vi "Process_TCP_Host.vi"(0 "Q_TCP_Cmd_IN":refnum<queue>, 1 "Q_TCP_Cmd_Err_IN":errorcluster, 2 "Q_GetPacket_IN":refnum<queue>, 3 "Q_GetPacket_Err_IN":errorcluster, 4 "Notifier_IN":refnum<notifier>, 5 "Notifier_Err_IN":errorcluster, 8 "PortNumber":u16=25534, 10 "IP Addr":string) -> (14 "Q_TCP_Cmd_OUT":refnum<queue>, 15 "Q_TCP_Cmd_Err_OUT":errorcluster, 16 "Q_GetPacket_OUT":refnum<queue>, 17 "Q_GetPacket_Err_OUT":errorcluster)   [LabVIEW 2023]
uses:
  HOST_GLOBAL.vi
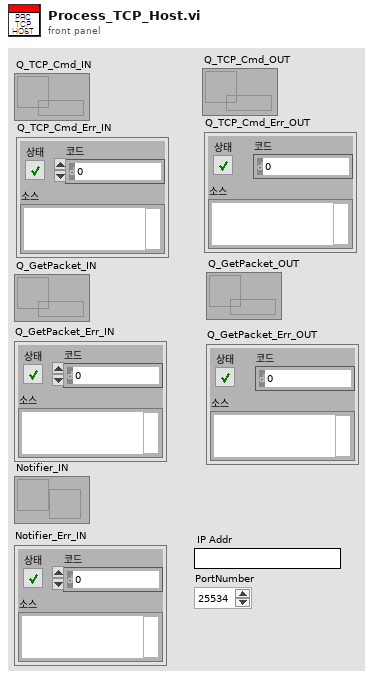
[diagram p1: front panel]
types:
  T1 = enum16{"Standard", "Buffered", "CRLF", "Immediate"}
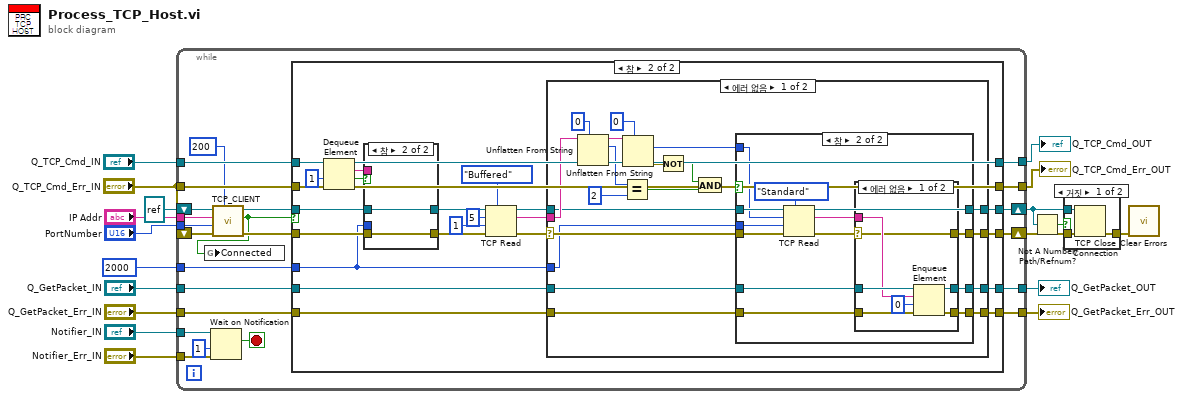
[diagram p0: block diagram]
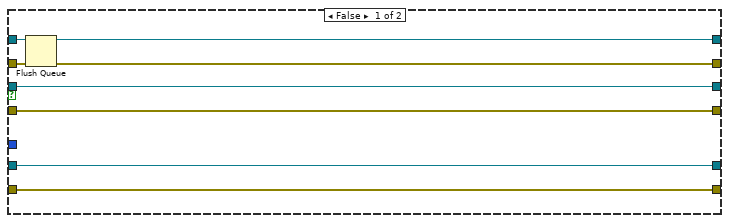
[diagram p3: hidden frame]
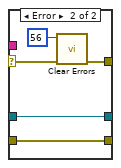
[diagram p5: hidden frame]
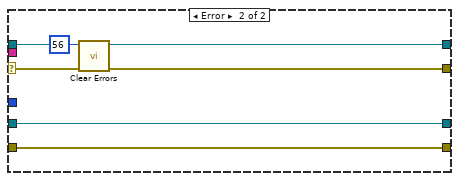
[diagram p6: hidden frame]
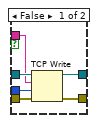
[diagram p7: hidden frame]
diagram:
  n1 = while {
    tunnel: "PortNumber" -> [w38]
    tunnel: "IP Addr" -> [w37]
    shift-right: [w23] -> w2
    shift-left: "Q_TCP_Cmd_Err_IN" -> [w41]
    shift-right: [w24] -> w1
    shift-left: refnum<k5> refnum ("TCP_Out") -> [w36]
    tunnel: "Q_TCP_Cmd_IN" -> [w35]
    tunnel: "Q_TCP_Cmd_Err_IN" -> [w34]
    tunnel: "Notifier_Err_IN" -> [w32]
    tunnel: "Notifier_IN" -> [w31]
    tunnel: 2000 ("타임아웃") -> [w29]
    tunnel: [w28] -> w9
    tunnel: [w27] -> w10
    tunnel: "Q_GetPacket_IN" -> [w26]
    tunnel: "Q_GetPacket_Err_IN" -> [w25]
    tunnel: [w22] -> w6
    tunnel: [w21] -> w5
    stop <- w19 stop-if-true
    n2 = Wait on Notification(notifier=w31, timeout in ms (-1)=1 ("타임아웃(ms) (-1)"), error in (no error)=w32) -> (notification=w19:bool)  [unwired: 1 in, 3 out]
    n3 = call "TCP_CLIENT.vi"("Timeout (ms)"=200, "Error In"=w41, "Port_Number"=w38, "IP_Address"=w37, "TCP_In"=w36) -> ("error out"=w40:errorcluster, "Connected?"=w30:bool, "TCP_Out"=w39:refnum<k5>)  [unwired: 4 in]
    n4 = global write "HOST_GLOBAL.vi" "Connected"(w30) -> ()
    n5 = case shown="참" w30 {
      tunnel: w40 -> [w48 w70]
      tunnel: w39 -> [w49 w69]
      tunnel: w35 -> [w47 w72]
      tunnel: w34 -> [w46 w71]
      tunnel: w29 -> [_ w56]
      tunnel: [w45 w66] -> w28
      tunnel: [w44 w65] -> w27
      tunnel: w26 -> [w42 w55]
      tunnel: w25 -> [w43 w54]
      tunnel: [w49 w53] -> w24
      tunnel: [w48 w52] -> w23
      tunnel: [w43 w50] -> w22
      tunnel: [w42 w51] -> w21
      frame False {
        n6 = Flush Queue(queue=w47, error in (no error)=w46) -> (queue out=w45:refnum<queue>, error out=w44:errorcluster)  [unwired: 1 out]
      }
      frame True {
        n7 = Dequeue Element(queue=w72, timeout in ms (-1)=1 ("타임아웃(ms) (-1)"), error in (no error)=w71) -> (queue out=w66:refnum<queue>, element=w68:string, timed out?=w67:bool, error out=w65:errorcluster)
        n8 = case shown="참" w67 {
          tunnel: w69 -> [w135 w137]
          tunnel: w70 -> [w134 w136]
          tunnel: [w133 w137] -> w61
          tunnel: [w132 w136] -> w60
          tunnel: w68 -> [w131 _]
          tunnel: w56 -> [w130 _]
          frame False {
            n9 = TCP Write(connection ID=w135, data in=w131, error in (no error)=w134, 9:w130) -> (connection ID out=w133:refnum<k5>, error out=w132:errorcluster)  [unwired: 1 out]
          }
          frame True {
          }
        }
        n10 = TCP Read(connection ID=w61, bytes to read=5 ("읽을 바이트"), error in (no error)=w60, 7:T1."Buffered" ("모드(standard)"), 9:1 ("타임아웃 ms (25000)")) -> (connection ID out=w58:refnum<k5>, data out=w57:string, error out=w59:errorcluster)
        n11 = case shown="에러 없음" w59 {
          selector: w59 -> [w82 w128]
          tunnel: [w79 w127] -> w52
          tunnel: w58 -> [w84 w126]
          tunnel: w57 -> [w85 _]
          tunnel: w56 -> [w80 _]
          tunnel: [w78 w126] -> w53
          tunnel: w55 -> [w77 w125]
          tunnel: w54 -> [w76 w124]
          tunnel: [w75 w125] -> w51
          tunnel: [w74 w124] -> w50
          frame No Error {
            n12 = Unflatten From String(type=i8 0, binary string=w85) -> (rest of the binary string=w88:string, value=w90:i8, error out=w87:errorcluster)  [unwired: 3 in]
            n13 = Equal?(x=w90, y=i8 2) -> (x = y?=w92:bool)
            n14 = Unflatten From String(type=0, binary string=w88, error in (no error)=w87) -> (value=w81:i32, error out=w93:errorcluster)  [unwired: 2 in, 1 out]
            n15 = Not(x=w93) -> (.not. x?=w94:bool)
            n16 = And(x=w94, y=w92) -> (x .and. y?=w83:bool)
            n17 = case shown="참" w83 {
              tunnel: w84 -> [w97 w111]
              tunnel: w82 -> [w98 w110]
              tunnel: w81 -> [_ w109]
              tunnel: w80 -> [_ w108]
              tunnel: [w98 w101] -> w79
              tunnel: [w97 w106] -> w78
              tunnel: w77 -> [w96 w105]
              tunnel: w76 -> [w95 w104]
              tunnel: [w96 w100] -> w75
              tunnel: [w95 w99] -> w74
              frame False {
              }
              frame True {
                n18 = TCP Read(connection ID=w111, bytes to read=w109, error in (no error)=w110, 7:T1."Standard" ("모드(standard)"), 9:w108) -> (connection ID out=w106:refnum<k5>, data out=w103:string, error out=w102:errorcluster)
                n19 = case shown="에러 없음" w102 {
                  selector: w102 -> [w115 w123]
                  tunnel: w105 -> [w118 w120]
                  tunnel: w104 -> [w117 w119]
                  tunnel: w103 -> [w116 _]
                  tunnel: [w115 w122] -> w101
                  tunnel: [w113 w120] -> w100
                  tunnel: [w112 w119] -> w99
                  frame No Error {
                    n20 = Enqueue Element(queue=w118, element=w116, timeout in ms (-1)=0 ("타임아웃(ms) (-1)"), error in (no error)=w117) -> (queue out=w113:refnum<queue>, error out=w112:errorcluster)  [unwired: 1 out]
                  }
                  frame Error {
                    n21 = call <vilib>:"Clear Errors.vi"("error in (no error)"=w123, "specific error code to clear (0: all)"=56) -> ("error out"=w122:errorcluster)  [unwired: 4 in, 1 out]
                  }
                }
              }
            }
          }
          frame Error {
            n22 = call <vilib>:"Clear Errors.vi"("error in (no error)"=w128, "specific error code to clear (0: all)"=56) -> ("error out"=w127:errorcluster)  [unwired: 4 in, 1 out]
          }
        }
      }
    }
  }
  "Q_TCP_Cmd_OUT" <- w9
  "Q_TCP_Cmd_Err_OUT" <- w10
  "Q_GetPacket_OUT" <- w5
  "Q_GetPacket_Err_OUT" <- w6
  n23 = Not A Number/Path/Refnum?(number/path/refnum=w1) -> (NaN/Path/Refnum?=w4:bool)
  n24 = case shown="거짓" w4 {
    tunnel: w1 -> [w140 _]
    tunnel: w2 -> [w139 w141]
    tunnel: [w138 w141] -> w3
    frame False {
      n25 = TCP Close Connection(connection ID=w140, error in (no error)=w139) -> (error out=w138:errorcluster)  [unwired: 1 in, 1 out]
    }
    frame True {
    }
  }
  n26 = call <vilib>:"Clear Errors.vi"("error in (no error)"=w3) -> ()  [unwired: 5 in, 2 out]
